vi "FPGA-Main2.vi"() -> ()   [LabVIEW 2019]
uses:
  <vilib>/Platform/TimedLoop/XDataNode/timing_clust.ctl
  <vilib>/Platform/TimedLoop/XDataNode/nitl_modes.ctl
  <vilib>/Platform/TimedLoop/XDataNode/wakeup.ctl
  <vilib>/rvi/Analysis/measure/FFT/simModelSupport/niFPGA FFT Outside SCTL Sim Properties.ctl
  <vilib>/rvi/Analysis/measure/FFT/simModelSupport/niFPGA FFT Sim Types.ctl
  <vilib>/rvi/Analysis/measure/FFT/simModelSupport/niFpgaFFTSimArithmeticProperties.ctl
  <vilib>/rvi/Analysis/measure/FFT/simModelSupport/niFpgaFFTSimDfxp.ctl
  <vilib>/fxp/LVFixedPointQuantizationPolicyTypeDef.ctl
  <vilib>/rvi/Analysis/measure/FFT/simModelSupport/niFPGA FFT Sim Properties.ctl
  <vilib>/rvi/Emulation/niFpgaGetClockAttributes.vi
  <vilib>/rvi/Emulation/niFpgaSctlEmulationGetInTimedLoop.vi
  <vilib>/rvi/Emulation/niFpgaEmulationReportErrorSimple.vi
  <vilib>/rvi/eio/common/nirviEmuTemplateMethod_errors.vi
  <vilib>/rvi/Emulation/niFpgaEmulationIsFPGAContextNoSignature.vi
  <vilib>/rvi/errors/niFpgaSetErrorForExecOnDevCompSimple.vi
  <vilib>/rvi/eio/common/nirviEmuReportErrorAndStop.vi
  <vilib>/rvi/DataTransferAndStorage/Container/Common/niFpgaContainerGetUniqueNameForEmu.vi
  <vilib>/rvi/FIFO/Fifo_Resource/nirvififoEmulationSetSize.vi
  <vilib>/rvi/FIFO/Fifo_Resource/nirviFifoEmulationQueueMgr.vi
  <instcachedir>/0/nirviFifoEmulationQueueMgr_E5CAEC123FF24DC58D834DCA3CDAA9B5.lvgen/nirviFifoEmulationQueueMgr_E5CAEC123FF24DC58D834DCA3CDAA9B5_006.vi
  <vilib>/rvi/FIFO/Fifo_Resource/nirvififoEmulationDetermineInputValidOut.vi
  <vilib>/rvi/FIFO/Fifo_Resource/nirvififoEmulationCreateLock.vi
  <vilib>/rvi/Emulation/niFpgaProcessEmulError.vi
  <vilib>/rvi/FIFO/Fifo_Resource/nirvififoEmulationObtainLock.vi
  <vilib>/rvi/FIFO/Fifo_Resource/nirvififoEmulationReleaseLock.vi
  <vilib>/rvi/occurrence/nirviWaitOnOccurrenceBase.vi
  <vilib>/rvi/errors/nirviReportUnexpectedCaseInternalError.vi
  <vilib>/rvi/errors/nirviReportUnexpectedCaseInternalError (U32).vi
  <vilib>/rvi/Emulation/niFpgaCriticalErrorInLSC.vi
  <vilib>/Utility/error.llb/Clear Errors.vi
  <vilib>/rvi/Analysis/measure/FFT/simModelSupport/niFpgaFFTSimModelOutsideSCTLCore.vi
  <vilib>/rvi/interface/RandomDataEmulation/nirviRandomDataMultiElementFPGAFIFO.vi
  <instcachedir>/0/nirviRandomDataMultiElementFPGAFIFO_1ED88BA00AC641F388A9B1FAA20E354D.lvgen/nirviRandomDataMultiElementFPGAFIFO_1ED88BA00AC641F388A9B1FAA20E354D_003.vi
  <vilib>/rvi/interface/RandomDataEmulation/niFpgaRandomDataHandleErrors.vi
  <vilib>/rvi/Analysis/measure/FFT/simModelSupport/niFpgaFFTSimModelCore.vi
  <vilib>/eio/EIONode/EIONode.xnode
  <vilib>/rvi/DataTransferAndStorage/Container/XNode/niFpgaContainer.xnode
  <vilib>/rvi/FIFO/Fifo_Resource/nirvififoEmulationWrite.vi
  <vilib>/rvi/FIFO/Fifo_Resource/nirvififoEmulationRead.vi
  <vilib>/rvi/Analysis/measure/FFT/XNode/niFpgaFFT.xnode
  <vilib>/rvi/interface/RandomDataEmulation/nirviRandomDataFpgaMultiElementTemplate.vi
  <vilib>/rvi/Analysis/measure/butterworth/XNode/niFpgaButterworthFilter.xnode
  <vilib>/rvi/interface/RandomDataEmulation/nirviRandomDataFpgaReadWriteTemplate.vi
  <vilib>/Platform/TimedLoop/XDataNode/XDataNode.xnode
  <vilib>/Platform/TimedLoop/XDataNode/XDNodeRunTimeDep.lvlib
panel:
  out "超时？ 5":bool
  out "超时？ 4":bool
  out "超时？ 3":bool
  out "超时？ 2":bool
  out "超时？":bool
  in  "Count(uSec)":u32=10 caption="计数器(uSec)"
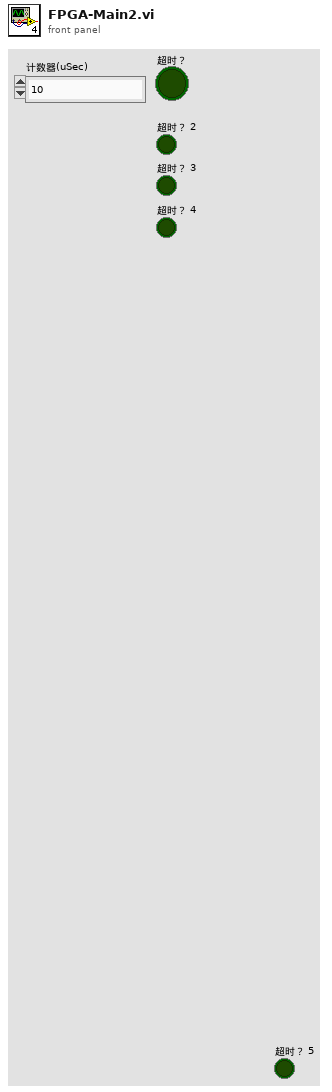
[diagram p1: front panel]
types:
  T1 = typedef "XDNodeRunTimeDep.lvlib/timing_clust.ctl" = cluster{"Expected End [f-1]":u64, "Actual End [f-1]":u64, "Finished Late? [f-1]":bool, "Expected End [i-1]":u64, "Actual End [i-1]":u64, "Finished Late? [i-1]":bool, "Expected Start [i]":u64, "Actual Start [i]":u64, "Expected Start [f]":u64, "Actual Start [f]":u64, "Source Name":string, "Structure Name":string, "Period":i64, "Deadline":i64, "Offset":i64, "Start":i64, "Priority":i32, "Timeout":i32, "Mode":T2, "Wakeup Reason":T3, "Error":errorcluster, "Source Type":string, "Secondary Source Type":string, "Global End Time":u64, "Global Start Time":u64, "Frame Duration":u64, "Iteration Duration":u64, "Assigned CPU":i32, "I/O Scan Engine Mode":u32}
  T2 = typedef "XDNodeRunTimeDep.lvlib/nitl_modes.ctl" = enum32{"No Change", "Process missed periods, maintain original phase", "Discard missed periods, maintain original phase", "Process missed periods, ignore original phase", "Discard missed periods, ignore original phase"}
  T3 = typedef "XDNodeRunTimeDep.lvlib/wakeup.ctl" = enum32{"Normal", "Aborted", "Asynchronous wakeup", "Timing source error", "Timed loop error", "Timeout"}
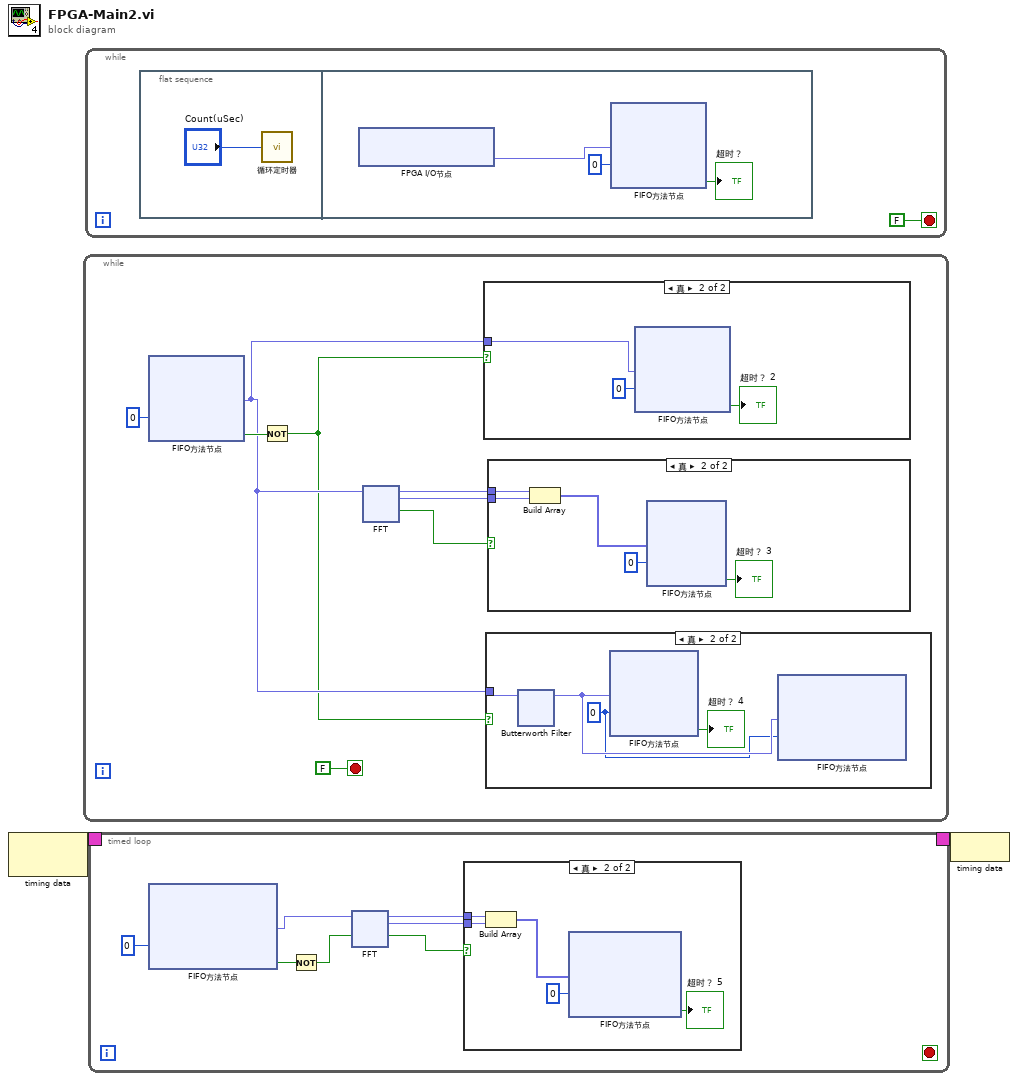
[diagram p0: block diagram]
diagram:
  n1 = node-c288() -> (w2:T1)  [unwired: 1 in]
  n2 = while {
    stop <- FALSE stop-if-true
    n3 = xnode ("FIFO方法节点")("超时"=0) -> ("元素"=w8:fxp<+/-,24,5>, "超时？"=w9:bool)  [unwired: 1 in, 1 out]
    n4 = Not(x=w9) -> (.not. x?=w7:bool)
    n5 = xnode "FFT"("实数数据输入"=w8) -> ("实数数据输出"=w5:fxp<+/-,32,14>, "虚数数据输出"=w4:fxp<+/-,32,14>, "输出有效"=w6:bool)  [unwired: 2 in, 1 out]
    n6 = case shown="真" w7 {
      tunnel: w8 -> [_ w50]
      frame False {
      }
      frame True {
        n7 = xnode ("FIFO方法节点")("元素"=w50, "超时"=0) -> ("超时？"=→"超时？ 2":bool)  [unwired: 1 in, 1 out]
      }
    }
    n8 = case shown="真" w7 {
      tunnel: w8 -> [_ w39]
      frame False {
      }
      frame True {
        w36 = 0 ("超时")
        n9 = xnode "Butterworth Filter"("输入数据"=w39) -> ("输出数据"=w37:fxp<+/-,24,5>)  [unwired: 2 in]
        n10 = xnode ("FIFO方法节点")("元素"=w37, "超时"=w36) -> ("超时？"=→"超时？ 4":bool)  [unwired: 1 in, 1 out]
        n11 = xnode ("FIFO方法节点")("元素"=w37, "超时"=w36) -> ()  [unwired: 1 in, 2 out]
      }
    }
    n12 = case shown="真" w6 {
      tunnel: w5 -> [_ w15]
      tunnel: w4 -> [_ w14]
      frame False {
      }
      frame True {
        n13 = Build Array(w15, w14) -> (w13:fxp<+/-,32,14>[])
        n14 = xnode ("FIFO方法节点")("元素"=w13, "超时"=0) -> ("超时？"=→"超时？ 3":bool)  [unwired: 1 in, 1 out]
      }
    }
  }
  n15 = while {
    stop <- FALSE stop-if-true
    n16 = flat-sequence {
      frame #0 {
        n17 = call "循环定时器"("Count(uSec)"="Count(uSec)") -> ()  [unwired: 1 out]
      }
      frame #1 {
        n18 = xnode "FPGA I/O节点"() -> ("ConnectorB/AI0"=w54:fxp<+/-,24,5>)  [unwired: 1 in, 1 out]
        n19 = xnode ("FIFO方法节点")("元素"=w54, "超时"=0) -> ("超时？"=→"超时？":bool)  [unwired: 1 in, 1 out]
      }
    }
  }
  n20 = timed-loop {
    timing: w2 -> [_]
    timing-out: [_] -> w1
    stop <- _ stop-if-true
    n21 = xnode ("FIFO方法节点")("超时"=0) -> ("元素"=w57:fxp<+/-,24,5>, "超时？"=w61:bool)  [unwired: 1 in, 1 out]
    n22 = Not(x=w61) -> (.not. x?=w56:bool)
    n23 = xnode "FFT"("实数数据输入"=w57, "输入有效"=w56) -> ("实数数据输出"=w59:fxp<+/-,32,14>, "虚数数据输出"=w58:fxp<+/-,32,14>, "输出有效"=w60:bool)  [unwired: 3 in, 2 out]
    n24 = case shown="真" w60 {
      tunnel: w59 -> [_ w64]
      tunnel: w58 -> [_ w63]
      frame False {
      }
      frame True {
        n25 = Build Array(w64, w63) -> (w67:fxp<+/-,32,14>[])
        n26 = xnode ("FIFO方法节点")("元素"=w67, "超时"=0) -> ("超时？"=→"超时？ 5":bool)  [unwired: 1 in, 1 out]
      }
    }
  }
  n27 = node-c288(w1) -> ()
